vi "direccionPieza.vi"(2 "posicion":i32[](array[numeric]), 3 "matrizPosiciones":i32[][](array[numeric])) -> (0 "Posicion":i32, 1 "Torre":i8)   [LabVIEW 2020]
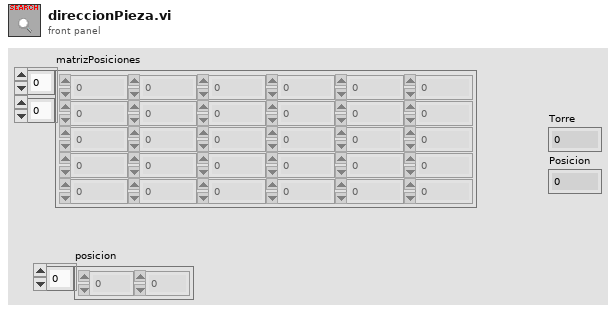
[diagram p1: front panel]
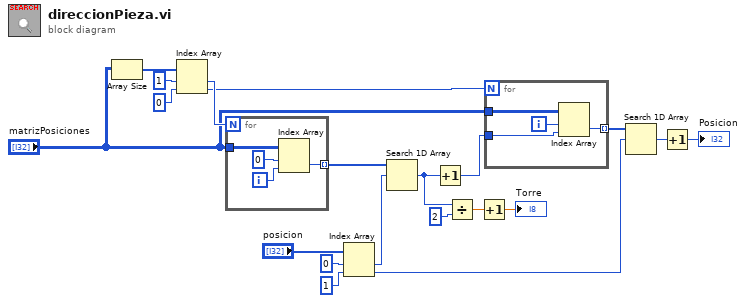
[diagram p0: block diagram]
diagram:
  n1 = Array Size(array="matrizPosiciones") -> (size(s)=w17:i32[])
  n2 = Index Array(array=w17, index #1=1 ("index"), index #2=0 ("index")) -> (element #1=w15:i32, element #2=w8:i32)
  n3 = for {
    N: w15 -> [_]
    tunnel: "matrizPosiciones" -> [w24]
    tunnel: [w21] -> w14 mode=indexing
    i -> [w22]
    n4 = Index Array(array=w24, index (row)=0, index (col)=w22) -> (element=w21:i32)
  }
  n5 = Index Array(array="posicion", index #1=0 ("index"), index #2=1 ("index")) -> (element #1=w13:i32, element #2=w4:i32)
  n6 = Search 1D Array(1D array=w14, element=w13) -> (index of element=w6:i32)  [unwired: 1 in]
  n7 = Increment(x=w6) -> (x+1=w1:i32)
  n8 = Divide(x=w6, y=2) -> (x/y=w11:dbl)
  n9 = Increment(x=w11) -> (x+1=→"Torre":dbl)
  n10 = for {
    N: w8 -> [_]
    tunnel: "matrizPosiciones" -> [w28]
    tunnel: [w27] -> w5 mode=indexing
    tunnel: w1 -> [w25]
    i -> [w26]
    n11 = Index Array(array=w28, index (row)=w26, index (col)=w25) -> (element=w27:i32)
  }
  n12 = Search 1D Array(1D array=w5, element=w4) -> (index of element=w3:i32)  [unwired: 1 in]
  n13 = Increment(x=w3) -> (x+1=→"Posicion":i32)
